vi "example_application.vi"() -> ()   [LabVIEW 2023]
uses:
  ctl_tdms.ctl
  ctl_structure_type.ctl
panel:
  in  "data":T1
  in  "apply":bool
  in  "Stop":bool
  out "error out":errorcluster
  in  "action":T2=enum."close"
  # "simple app to see how the data is structured in the TDMS; for 2 data channels\nThis is valid for \"Decimate\" setting. If you use 'Interleaved' you'll have to remove the 2D transpose in the code"
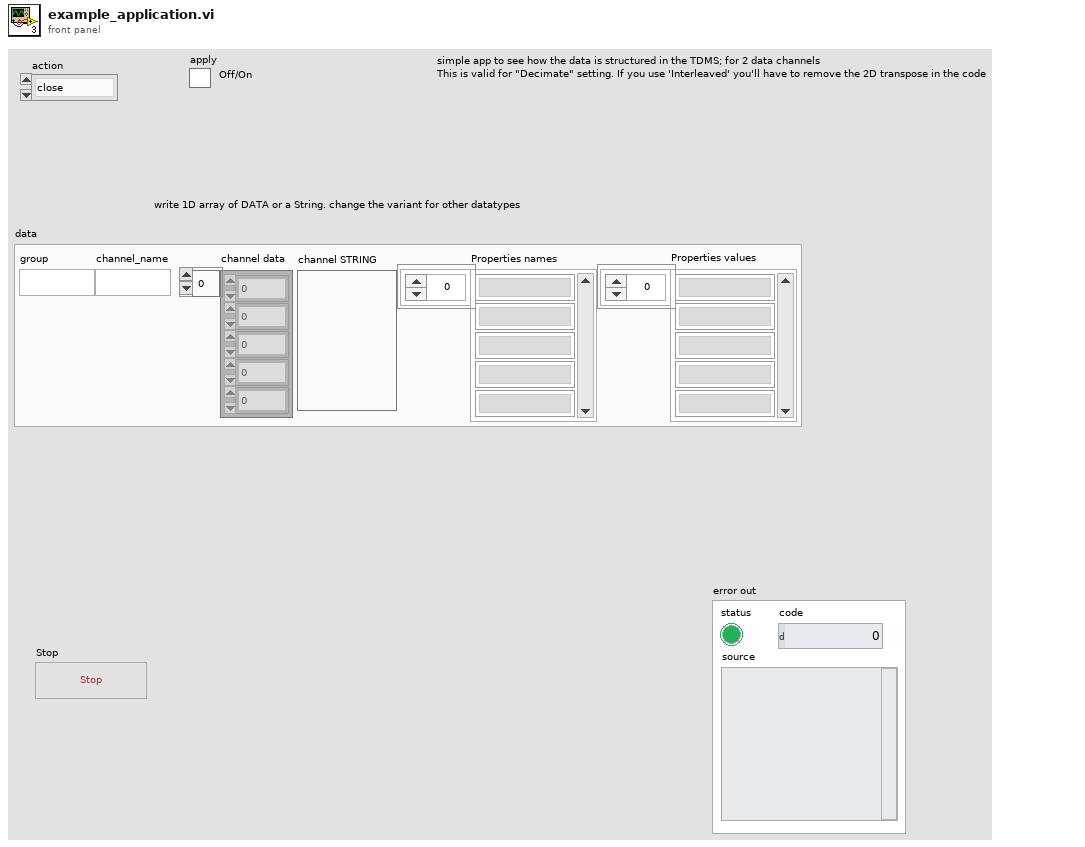
[diagram p1: front panel]
types:
  T1 = typedef "ctl_structure_type.ctl" = cluster{"group":string, "channel_name":string, "channel data":dbl[], "channel STRING":string, "Properties names":string[], "Properties values":string[]}
  T2 = typedef "ctl_tdms.ctl" = enum16{"create", "write_text", "write", "close"}
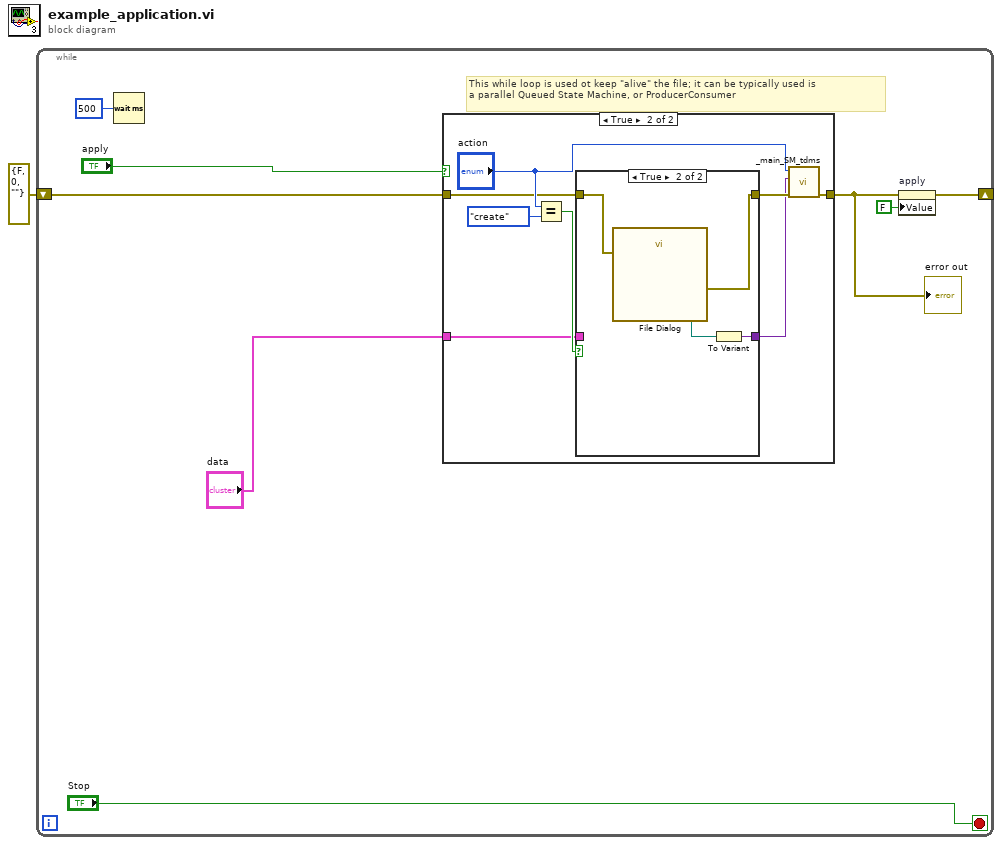
[diagram p0: block diagram]
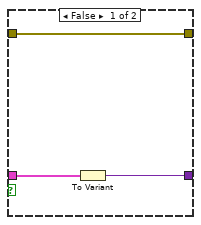
[diagram p3: hidden frame]
diagram:
  n1 = while {
    shift-right: [w4] -> _
    shift-left: errorcluster {"status"=FALSE, "code"=0, "source"=""} ("error in") -> [w5]
    stop <- "Stop" stop-if-true
    # "This while loop is used ot keep \"alive\" the file; it can be typically used is\na parallel Queued State Machine, or ProducerConsumer"
    n2 = Wait (ms)(milliseconds to wait=u32 500) -> ()  [unwired: 1 out]
    n3 = case shown="True" "apply" {
      tunnel: [w10 w18] -> w2
      tunnel: w5 -> [w10 w14]
      tunnel: "data" -> [_ w11]
      frame False {
      }
      frame True {
        n4 = Equal?(x="action", y=ctl_tdms."create") -> (x = y?=w15:bool)
        n5 = case shown="True" w15 {
          tunnel: w14 -> [w21 w25]
          tunnel: [w21 w24] -> w13
          tunnel: [w19 w22] -> w12
          tunnel: w11 -> [w20 _]
          frame False {
            n6 = To Variant(anything=w20) -> (Variant=w19:variant)
          }
          frame True {
            n7 = call "File Dialog"("error in"=w25) -> ("selected path"=w23:path, "error out"=w24:errorcluster)  [unwired: 11 in, 2 out]
            n8 = To Variant(anything=w23) -> (Variant=w22:variant)
          }
        }
        n9 = call "_main_SM_tdms.vi"("error in"=w13, "Variant"=w12, "Enum"="action") -> ("error out"=w18:errorcluster)  [unwired: 8 in]
      }
    }
    "error out" <- w2
    n10 = property on="apply" class="Bool (strict)"(error in=w2, "Value"=FALSE ("apply")) -> (error out=w4:errorcluster)  [unwired: 1 in, 1 out]
  }
